vi "CSM to check message.vi"() -> ()   [LabVIEW 2014]
uses:
  user.lib/_NEVSTOP/Communicable State Machine(CSM)/_Support/Priority Queue/Priority Queue.lvclass/Priority Queue.ctl
  user.lib/_NEVSTOP/Communicable State Machine(CSM)/_Support/Process/CSMP-Async Call.vi
  user.lib/_NEVSTOP/Communicable State Machine(CSM)/_Support/GlobalEvent/GEvt-Generate Status Log.vi
  user.lib/_NEVSTOP/Communicable State Machine(CSM)/_Support/Process/CSMP-Broadcast.vi
  user.lib/_NEVSTOP/Communicable State Machine(CSM)/_Support/GlobalEvent/GEvt-Generate Interrupt Log.vi
  user.lib/_NEVSTOP/Communicable State Machine(CSM)/_Support/GlobalEvent/GEvt-Generate Register Log.vi
  user.lib/_NEVSTOP/Communicable State Machine(CSM)/_Support/Process/CSMP-Register Status.vi
  user.lib/_NEVSTOP/Communicable State Machine(CSM)/_Support/GlobalEvent/GEvt-Generate Unregister Log.vi
  user.lib/_NEVSTOP/Communicable State Machine(CSM)/_Support/Process/CSMP-Unregister Status.vi
  user.lib/_NEVSTOP/Communicable State Machine(CSM)/_Support/Process/CSMP-Sync Call.vi
  user.lib/_NEVSTOP/Communicable State Machine(CSM)/_Support/CSMQ/_CSMObj-Unlock.vi
  user.lib/_NEVSTOP/Communicable State Machine(CSM)/_Support/Process/CSMP-PostPostMsg.vi
  user.lib/_NEVSTOP/Communicable State Machine(CSM)/_Support/Process/CSMP-PostSendMsg.vi
  user.lib/_NEVSTOP/Communicable State Machine(CSM)/_Support/CSMQ/_CSMObj-Lock State.vi
  user.lib/_NEVSTOP/Communicable State Machine(CSM)/_Support/Common/Splite Reason String Part.vi
  user.lib/_NEVSTOP/Communicable State Machine(CSM)/_Support/Common/Trim Single line Text.vi
  user.lib/_NEVSTOP/Communicable State Machine(CSM)/_Support/CSMQ/_CSMOFGV Release.vi
  user.lib/_NEVSTOP/Communicable State Machine(CSM)/_Support/Common/Remove Comments from Line.vi
  user.lib/_NEVSTOP/Communicable State Machine(CSM)/_Support/Common/Splite Single-line Message.vi
  user.lib/_NEVSTOP/Communicable State Machine(CSM)/_Support/Common/Parse Next Single-line State.vi
  user.lib/_NEVSTOP/Communicable State Machine(CSM)/_Support/CSMQ/_CSMObj-Log Error if in a Remote Session.vi
  user.lib/_NEVSTOP/Communicable State Machine(CSM)/_Support/CSMQ/_CSMOFGV Obtain.vi
  user.lib/_NEVSTOP/Communicable State Machine(CSM)/_Support/GlobalEvent/GEvt-Generate State Change Log.vi
  user.lib/_NEVSTOP/Communicable State Machine(CSM)/_Support/GlobalEvent/GEvt-Generate Remaining States Log.vi
  user.lib/_NEVSTOP/Communicable State Machine(CSM)/_Support/GlobalEvent/GEvt-Generate Complete Log.vi
  user.lib/_NEVSTOP/Communicable State Machine(CSM)/AdvanceAPI/CSM - Revert Arguments-Safe String.vi
  user.lib/_NEVSTOP/Communicable State Machine(CSM)/_Support/CSMQ/_CSMObj-Message Check.vi
  user.lib/_NEVSTOP/Communicable State Machine(CSM)/_Support/FGV-BroadcastRegistry/Cache-Broadcast Registry Search Result.vi
  user.lib/_NEVSTOP/Communicable State Machine(CSM)/AdvanceAPI/CSM - Register Status Change.vi
  user.lib/_NEVSTOP/Communicable State Machine(CSM)/AdvanceAPI/CSM - Unregister Status Change.vi
  user.lib/_NEVSTOP/Communicable State Machine(CSM)/Utility/uuid.vi
  user.lib/_NEVSTOP/Communicable State Machine(CSM)/_Support/Common/CSM-Name to CSM-Mode.vi
  user.lib/_NEVSTOP/Communicable State Machine(CSM)/_Support/Priority Queue/Not a Refnum.vi
  user.lib/_NEVSTOP/Communicable State Machine(CSM)/AdvanceAPI/CSM - Keywords.vi
  user.lib/_NEVSTOP/Communicable State Machine(CSM)/_Support/GlobalEvent/FGV-GlobalEventRef.vi
  user.lib/_NEVSTOP/Communicable State Machine(CSM)/_Support/CSMQ/_CSMOFGV.vi
  user.lib/_NEVSTOP/Communicable State Machine(CSM)/_Support/CSMQ/_CSMOFGV Dequeue.vi
  user.lib/_NEVSTOP/Communicable State Machine(CSM)/_Support/CSMQ/_CSMObj-Enqueue Cross-Module Message.vi
  user.lib/_NEVSTOP/Communicable State Machine(CSM)/_Support/GlobalEvent/FGV-StatusChangeEventRef.vi
  user.lib/_NEVSTOP/Communicable State Machine(CSM)/_Support/FGV-BroadcastRegistry/global-Broadcast Cache Change Flag.vi
  user.lib/_NEVSTOP/Communicable State Machine(CSM)/_Support/FGV-BroadcastRegistry/FGV-BroadcastRegistry.vi
  user.lib/_NEVSTOP/Communicable State Machine(CSM)/Communicable State Machine.lvlib
panel:
  in  "DoSth: DoB -@ CSM":bool
  in  "DoSth: DoB -> CSM":bool
  in  "DoSth: DoA -@ CSM":bool
  in  "DoSth: DoA -> CSM":bool
  in  "API: API2 -@ CSM":bool
  in  "API: API2 -> CSM":bool
  in  "API: API1 -@ CSM":bool
  in  "API: API1 -> CSM":bool
  out "State History":string
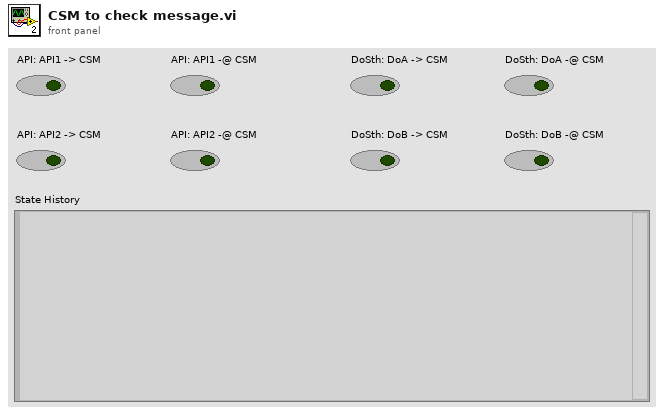
[diagram p1: front panel]
types:
  T1 = enum32{"Invalid", "Standard", "Closed", "Hidden", "Minimized", "Maximized"}
  T2 = enum32{"invalid app kind", "Development System", "Run Time System", "Student Edition", "Embedded LabVIEW", "Evaluation", "Custom"}
  T3 = typedef "Communicable State Machine.lvlib/_CSM_Response Source Message.ctl" = cluster{"‘State":string, "’Arguments":string, "’Error":errorcluster}
  T4 = cluster{"Core":cluster{"Current VI Reference":refnum<vi>, "Close Panel on Exit?":bool}, "Your Boolean data":bool, "Your string data":string}
  T5 = cluster{"Current VI Reference":refnum<vi>, "Close Panel on Exit?":bool}
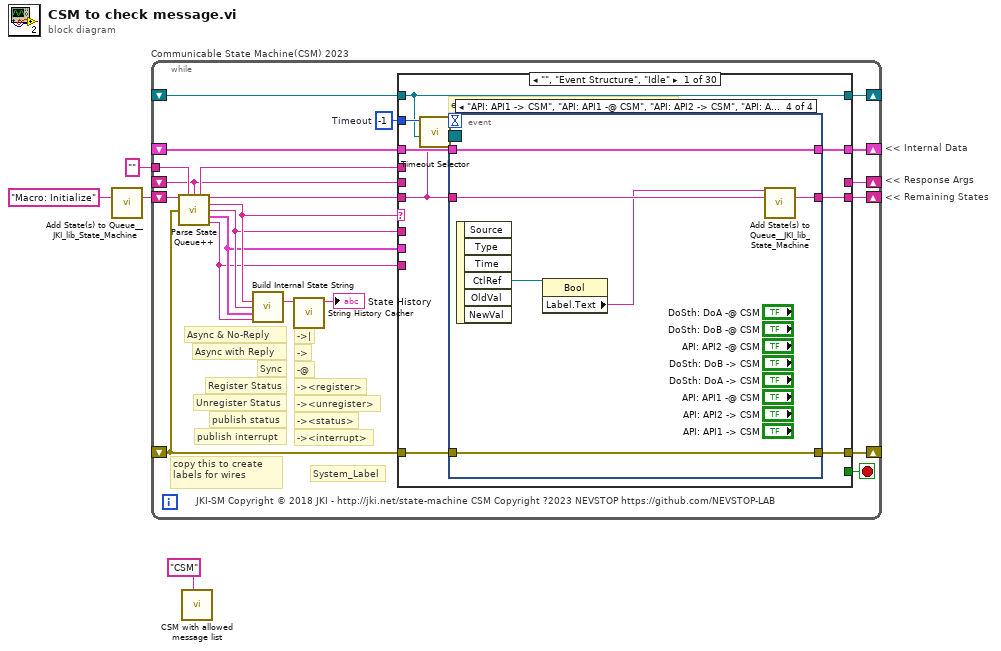
[diagram p0: block diagram]
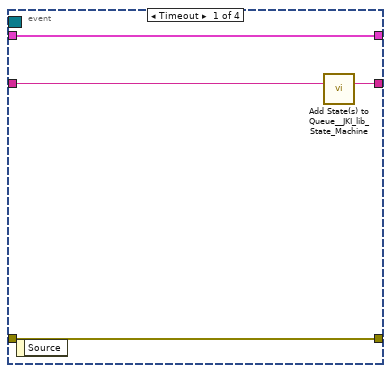
[diagram p2: hidden frame]
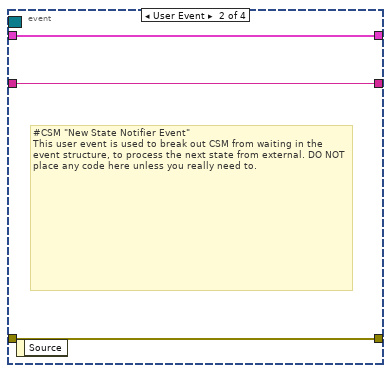
[diagram p3: hidden frame]
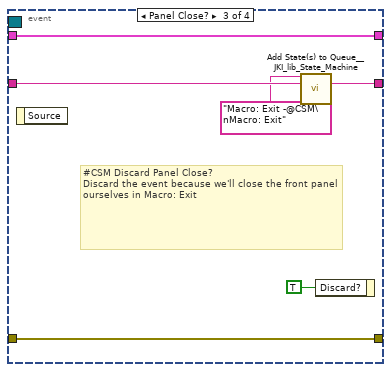
[diagram p4: hidden frame]
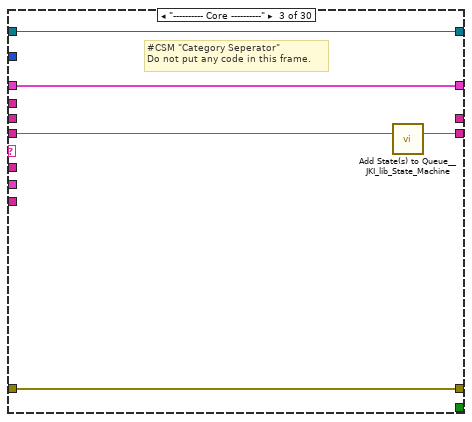
[diagram p6: hidden frame]
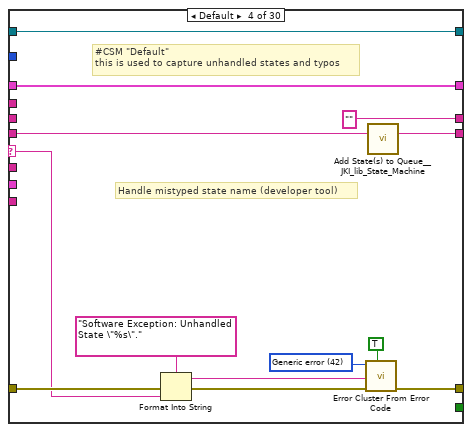
[diagram p7: hidden frame]
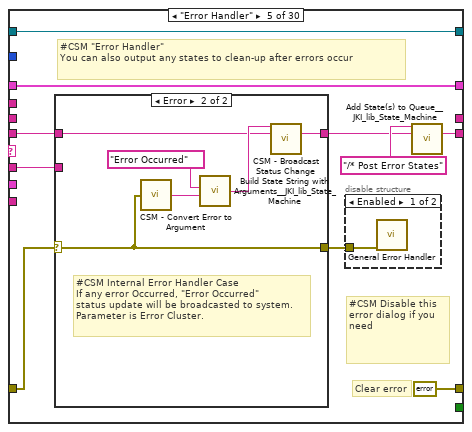
[diagram p8: hidden frame]
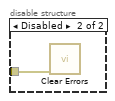
[diagram p9: hidden frame]
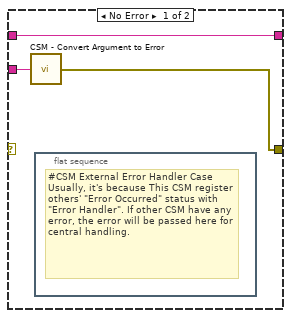
[diagram p10: hidden frame]
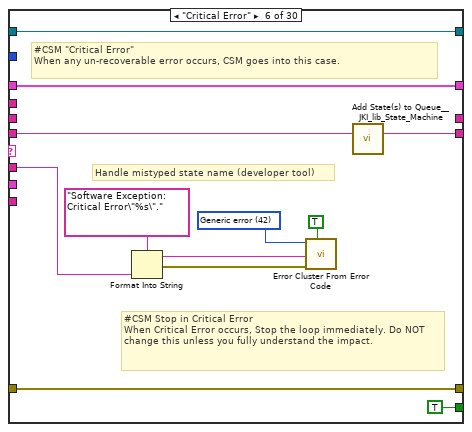
[diagram p11: hidden frame]
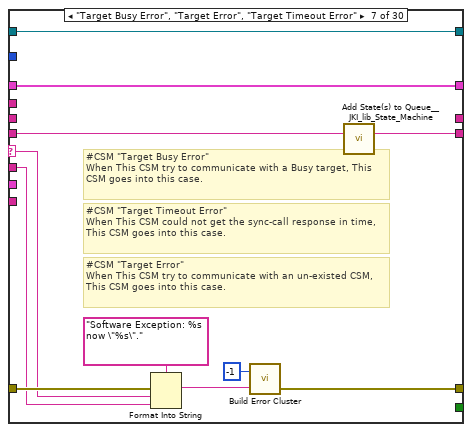
[diagram p12: hidden frame]
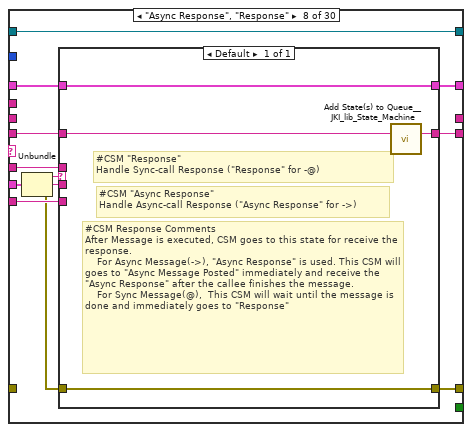
[diagram p13: hidden frame]
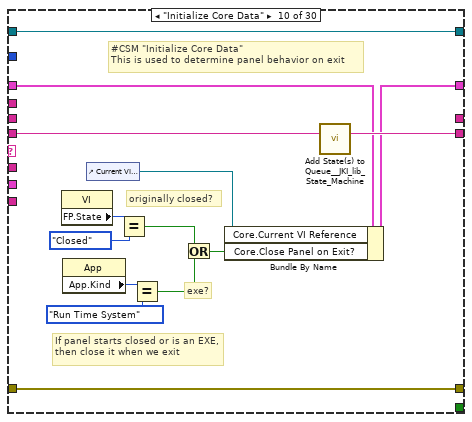
[diagram p15: hidden frame]
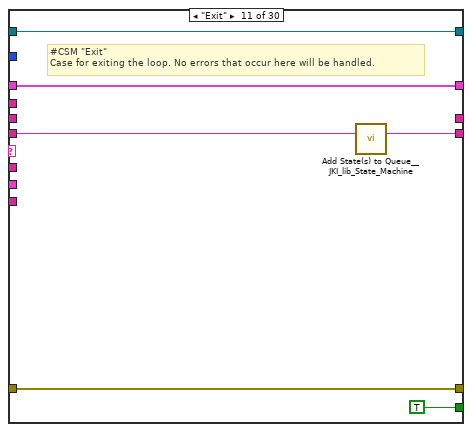
[diagram p16: hidden frame]
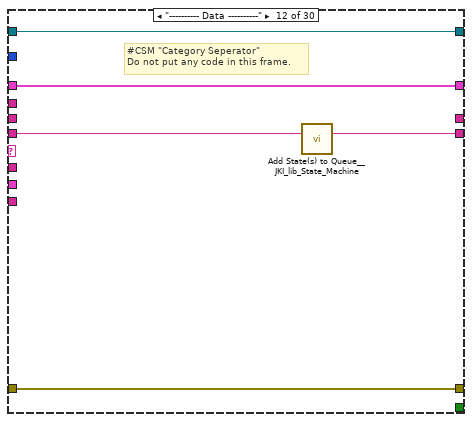
[diagram p17: hidden frame]
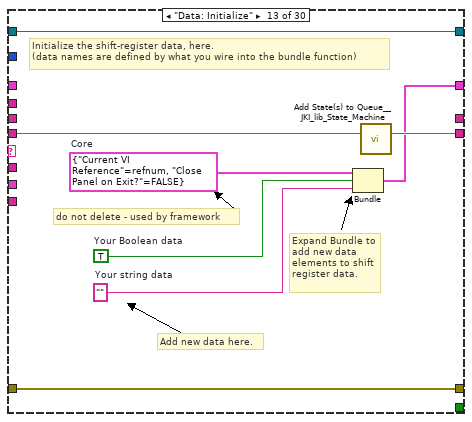
[diagram p18: hidden frame]
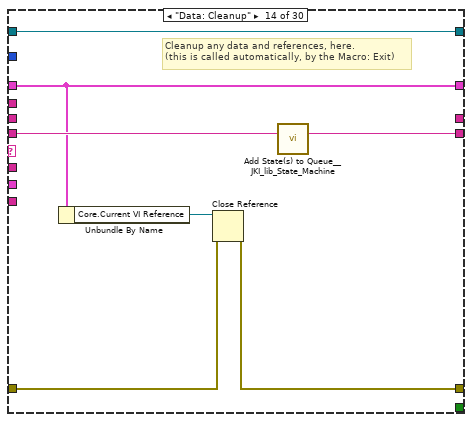
[diagram p19: hidden frame]
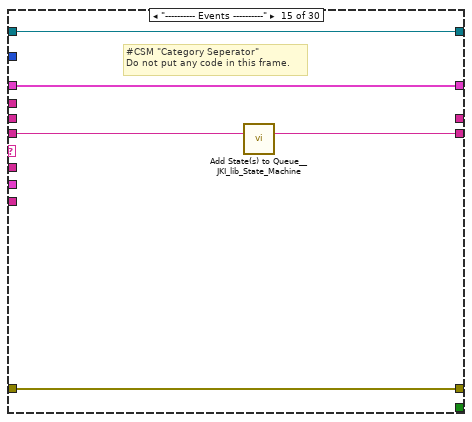
[diagram p20: hidden frame]
diagram:
  # "<< Internal Data"
  # "<< Response Args"
  # "<< Remaining States"
  n1 = call <vilib>:"Add State(s) to Queue__JKI_lib_State_Machine.vi"("State(s) in (\"\")"="Macro: Initialize" ("Init State(\"Macro: Initialize\")")) -> ("States Out"=w4:string)  [unwired: 14 in]
  n2 = while "Communicable State Machine(CSM) 2023" {
    shift-right: [w20] -> _
    shift-left: _ -> [w19]
    shift-right: [w23] -> _
    shift-left: _ -> [w17]
    shift-right: [w22] -> _
    shift-left: w4 -> [w24]
    tunnel: "" ("Name(\"\" to use uuid)") -> [w13]
    shift-right: [w16] -> _
    shift-left: _ -> [w5]
    shift-right: [w15] -> _
    shift-left: _ -> [w14]
    stop <- w21 stop-if-true
    w18 = -1  # Timeout
    # "-><interrupt>"
    # "-><status>"
    # "-><unregister>"
    # "-><register>"
    # "-@"
    # "->"
    # "->|"
    # "publish interrupt"
    # "publish status"
    # "Unregister Status"
    # "Register Status"
    # "Sync"
    # "Async with Reply"
    # "Async & No-Reply"
    # "copy this to create labels for wires"
    # "System_Label"
    # "JKI-SM Copyright © 2018 JKI - http://jki.net/state-machine CSM Copyright ?2023 NEVSTOP https://github.com/NEVSTOP-LAB"
    n3 = call "Parse State Queue++.vi"("State Queue"=w24, "Name(\"\" to use uuid)"=w13, "Response Arguments"=w5, "Error In (no error)"=w17) -> ("Name Used"=w6:string, "Remaining States"=w25:string, "Current State"=w10:string, "Arguments"=w9:string, ">> Response Source Message >>"=w8:T3, ">> Source CSM >>"=w7:string)  [unwired: 6 in]
    n4 = call "Build Internal State String.vi"("State"=w10, "Arguments (\"\")"=w9, ">> Response Source Message >>"=w8, "Source (\"\")"=w7) -> ("State with Arguments"=w11:string)  [unwired: 11 in]
    n5 = call "String History Cacher.vi"("String"=w11) -> ("String Cache"=→"State History":string)  [unwired: 10 in]
    n6 = case shown="\"\", \"Event Structure\", \"Idle\"" w10 {
      selector: w10 -> [_ _ _ w65 _ _ w112 _ _ _ _ _ _ _ _ _ _ _ _ _ _ _ _ _ _ _ _ _ _ _]
      tunnel: w25 -> [w26 w56 w62 w69 w80 w106 w114 w125 w138 w153 w159 w164 w172 w179 w184 w191 w195 w201 w206 w213 w229 w299 w305 w316 w319 w324 w330 w338 w344 w350]
      tunnel: w9 -> [_ _ _ _ w79 w99 w113 w124 _ _ _ _ _ _ _ _ _ _ _ w208 w223 _ _ _ _ _ w327 _ _ _]
      tunnel: w19 -> [w33 w55 w59 w67 w84 w107 w116 w127 w137 w146 w157 w161 _ w174 w181 w190 w194 w198 w204 w211 w225 w296 w302 w313 w318 w323 w329 w335 w341 w347]
      tunnel: [w32 w57 w60 w71 errorcluster {"status"=FALSE, "code"=0, "source"=""} ("error out") w108 w110 w130 w139 w150 w156 w162 w169 w175 w182 w185 w193 w199 w203 w209 w226 w297 w303 w314 w320 w325 w331 w336 w342 w348] -> w23
      tunnel: w17 -> [w31 w57 w60 w70 w81 w108 w118 _ w139 w150 w156 w162 w169 w176 w182 _ w196 w199 w203 w210 w227 w297 w303 w314 w320 w325 w331 w336 w342 w348]
      tunnel: [w34 w56 w61 w68 w76 w105 w117 w126 w138 w152 w158 w163 w171 w178 w183 w191 w195 w200 w205 w212 w228 w298 w304 w315 w319 w324 w330 w337 w343 w349] -> w22
      tunnel: [_ _ _ _ _ TRUE _ _ _ _ TRUE _ _ _ _ _ _ _ _ _ _ _ _ _ _ _ _ _ _ _] -> w21
      tunnel: [w30 w55 w59 w67 w84 w107 w116 w128 w137 w151 w157 w161 w170 w174 w181 w190 w194 w198 w204 w211 w225 w296 w302 w313 w318 w323 w329 w335 w341 w347] -> w20
      tunnel: w18 -> [w29 _ _ _ _ _ _ _ _ _ _ _ _ _ _ _ _ _ _ _ _ _ _ _ _ _ _ _ _ _]
      tunnel: w7 -> [_ _ _ _ _ _ _ w122 _ _ _ _ _ _ _ _ _ _ _ _ _ _ _ _ _ _ _ _ _ _]
      tunnel: w8 -> [_ _ _ _ _ _ _ w129 _ _ _ _ _ _ _ _ _ _ _ _ _ _ _ _ _ _ _ _ _ _]
      tunnel: [_ _ _ "" _ _ _ _ _ _ _ _ _ _ _ _ _ _ _ _ _ _ _ _ _ "API1 Response" w326 _ "DoA Finished" "DoB Finished"] -> w16
      tunnel: [w28 w54 w58 w63 w83 w97 w115 w131 w136 w140 w154 w160 w165 w173 w180 w189 w192 w197 w202 w207 w222 w295 w300 w306 w317 w322 w328 w334 w340 w346] -> w15
      tunnel: w14 -> [w28 w54 w58 w63 w83 w97 w115 w131 w136 w140 w154 w160 w165 w173 w180 _ w192 w197 w202 w207 w222 w295 w300 w306 w317 w322 w328 w334 w340 w346]
      tunnel: w6 -> [_ _ _ _ _ _ _ _ _ _ _ _ _ _ _ w188 _ _ _ _ _ _ _ _ _ _ _ _ _ _]
      tunnel: w5 -> [_ _ _ _ _ _ _ _ _ _ _ _ _ _ _ _ _ _ _ _ _ _ _ _ _ _ _ _ _ _]
      frame "", "Event Structure", "Idle" {
        # "executes when the state queue is empty"
        n7 = call "Timeout Selector.vi"("Remaining States"=w26, "Timeout Expected"=w29) -> ("Timeout"=w27:i32)  [unwired: 5 in]
        n8 = event shown="[3] \"API: API1 -> CSM\", \"API: API1 -@ CSM\", \"API: API2 -> CSM\", \"API: API2 -@ CSM\", \"DoSth: DoA -> CSM\", \"DoSth: DoA -@ CSM\", \"DoSth: DoB -> CSM\", \"DoSth: DoB -@ CSM\": Value Change" {
          selector: w28 -> [_ _ _ _]
          dyn-events: _ -> [_ _ _ _]
          timeout: w27 -> [_ _ _ _]
          tunnel: w26 -> [w38 w40 w47 w51]
          tunnel: [w37 w40 w46 w50] -> w34
          tunnel: w33 -> [w35 w41 w44 w52]
          tunnel: [w36 w39 w45 w53] -> w32
          tunnel: w31 -> [w36 w39 w45 w53]
          tunnel: [w35 w41 w44 w52] -> w30
          event Timeout {
            n9 = event-data() -> ()  [unwired: 1 in, 1 out]
            n10 = call <vilib>:"Add State(s) to Queue__JKI_lib_State_Machine.vi"("State(s) in (\"\")"=w38) -> ("States Out"=w37:string)  [unwired: 14 in]
          }
          event User Event {
            # "#CSM \"New State Notifier Event\"\nThis user event is used to break out CSM from waiting in the event structure, to process the next state from external. DO NOT place any code here unless you really need to."
            n11 = event-data() -> ()  [unwired: 1 in, 1 out]
          }
          event Panel Close? {
            # "#CSM Discard Panel Close?\nDiscard the event because we'll close the front panel ourselves in Macro: Exit"
            n12 = event-data() -> ()  [unwired: 1 in, 1 out]
            n13 = call <vilib>:"Add State(s) to Queue__JKI_lib_State_Machine.vi"("State(s) in Front (\"\")"="Macro: Exit -@CSM\nMacro: Exit", "State(s) in (\"\")"=w47) -> ("States Out"=w46:string)  [unwired: 13 in]
            n14 = event-data("Discard?"=TRUE) -> ()  [unwired: 1 in, 1 out]
          }
          event "API: API1 -> CSM", "API: API1 -@ CSM", "API: API2 -> CSM", "API: API2 -@ CSM", "DoSth: DoA -> CSM", "DoSth: DoA -@ CSM", "DoSth: DoB -> CSM", "DoSth: DoB -@ CSM": Value Change {
            n15 = event-data() -> ("CtlRef"=w49:refnum<vi>)  [unwired: 1 in, 5 out]
            n16 = property class="Bool"(reference=w49) -> ("Label.Text"=w48:string)  [unwired: 1 in, 2 out]
            n17 = call <vilib>:"Add State(s) to Queue__JKI_lib_State_Machine.vi"("State(s) in Front (\"\")"=w48, "State(s) in (\"\")"=w51) -> ("States Out"=w50:string)  [unwired: 13 in]
          }
        }
      }
      frame "CSM Documentation" {
        # "#CSM README FIRST\n\nCSM is a LabVIEW application framework that builds upon JKI State Machine (JKISM). It follows the pattern of JKISM and extends the keywords to describe message communication between CSM modules, including concepts such as Sync-Message, Async-Message, Subscription/Unsubscription of status - essential elements for creating reusable code modules. For more information, please visit the CSM wiki: https://github.com/NEVSTOP-LAB/JKI-State-Machine-Plus-Plus/wiki\n\nFor instructions on JKI State Machine, visit: http://jki.net/state-machine/\nFor information about CSM, visit: https://github.com/NEVSTOP-LAB"
        # "#CSM \"Documentation\"\nCase for holding CSM Documenation"
      }
      frame "---------- Core ----------" {
        # "#CSM \"Category Seperator\"\nDo not put any code in this frame."
        n18 = call <vilib>:"Add State(s) to Queue__JKI_lib_State_Machine.vi"("State(s) in (\"\")"=w62) -> ("States Out"=w61:string)  [unwired: 14 in]
      }
      frame Default {
        w74 = 42 items=["No error", "Argument error", "Memory is full", "Out of zone", "End of file", "File already open", "Generic file I/O error", "File not found", "File permission error", "Disk is full", "Duplicate path", "Too many files open", "System feature not enabled", "Resource file not found", "Cannot add resource", "Resource not found", "Image not found", "Image memory error", "Pen does not exist", "Config type invalid", "Config token not found", "Config parse error", "Config memory error", "Bad external code format", "Bad external code offset", "External code not present", "Null window", "Destroy window error", "Null menu", "Print aborted", "Bad print record", "Print driver error", "Windows error during printing", "Memory error during printing", "Print dialog error", "Generic print error", "Invalid device refnum", "Device not found", "Device parameter error", "Device unit error", "Cannot open device", "Device call aborted", "Generic error", "Cancelled by user", "Object ID too low", "Object ID too high", "Object not in heap", "Unknown heap", "Unknown object (invalid DefProc)", "Unknown object (DefProc not in table)", "Message out of range", "Invalid (null) method", "Unknown message", "Manager call not supported", "Bad address", "Network operation in progress", "Network operation timed out", "Connection is busy", "Network attribute not supported", "Network error", "Address in use", "System out of memory", "Connection aborted", "Connection refused", "Not connected", "Already connected", "Connection closed", "Initialization error (interapplication manager)", "Bad occurrence", "Wait on unbound occurrence handler", "Occurrence queue overflow", "Datalog type conflict", "Unused", "Unrecognized type (interapplication manager)", "Memory corrupt", "Failed to make temporary DLL", "Old CIN version", "Drag socket not found", "Failed to load drop-object", "Failed to register OLE object", "Failed to release OLE object", "Format specifier type mismatch", "Unknown format specifier", "Too few format specifiers", "Too many format specifiers", "Scan failed", "Newer CIN version", "Error converting to variant", "Runtime menu error", "Password tampered", "Variant attribute not found", "Incompatible variant data type", "Event data is not available", "Event Store is not present", "Occurrence is not found", "Event Queue is not created", "Event info is not available", "Refnum passed is NULL", "Error retrieving Class GUID", "Error retrieving CoClass GUID", "Error retrieving TypeLib GUID.", "Bad built application magic bytes.", "Specific driver is different from the specific driver associated with the Logical Name.", "There is no session opened to the class driver.", "Max Error", "MAX - Error with config objects", "MAX - Error loading configuration", "MAX - Group not supported"]
        # "#CSM \"Default\"\nthis is used to capture unhandled states and typos"
        # "Handle mistyped state name (developer tool)"
        n19 = Format Into String(format string="Software Exception: Unhandled State \"%s\"." ("message"), error in=w70, w65) -> (resulting string=w73:string, error out=w72:errorcluster)  [unwired: 1 in]
        n20 = call <vilib>:"Error Cluster From Error Code.vi"("show call chain? (False)"=TRUE, "error in (no error)"=w72, "error message (\"\")"=w73, "error code (0)"=w74) -> ("error out"=w71:errorcluster)  [unwired: 5 in]
        n21 = call <vilib>:"Add State(s) to Queue__JKI_lib_State_Machine.vi"("State(s) in (\"\")"=w69) -> ("States Out"=w68:string)  [unwired: 14 in]
      }
      frame "Error Handler" {
        # "#CSM Disable this error dialog if you need"
        # "#CSM \"Error Handler\"\nYou can also output any states to clean-up after errors occur"
        # "Clear error"
        n22 = case shown="Error" w81 {
          selector: w81 -> [_ w91]
          tunnel: [w90 w93] -> w77
          tunnel: w80 -> [w90 w92]
          tunnel: w79 -> [w89 _]
          tunnel: [w88 w91] -> w82
          frame No Error {
            n23 = call "CSM - Convert Argument to Error.vi"("Argument"=w89) -> ("error"=w88:errorcluster)  [unwired: 4 in]
            n24 = flat-sequence {
              frame #0 {
                # "#CSM External Error Handler Case\nUsually, it's because This CSM register others' \"Error Occurred\" status with \"Error Handler\". If other CSM have any error, the error will be passed here for central handling."
              }
            }
          }
          frame Error {
            # "#CSM Internal Error Handler Case \nIf any error Occurred, \"Error Occurred\" \nstatus update will be broadcasted to system.\nParameter is Error Cluster."
            n25 = call "CSM - Convert Error to Argument.vi"("error in (no error)"=w91) -> ("Arguments"=w95:string)  [unwired: 4 in]
            n26 = call <vilib>:"Build State String with Arguments__JKI_lib_State_Machine.vi"("Arguments (\"\")"=w95, "State"="Error Occurred" ("Status with Arguments")) -> ("State with Arguments"=w94:string)  [unwired: 4 in]
            n27 = call "CSM - Broadcast Status Change.vi"("Status with Arguments"=w94, "State Queue"=w92) -> ("Remaining States"=w93:string)  [unwired: 13 in]
          }
        }
        n28 = disable-structure shown="Enabled" {
          disable-tunnel: w82 -> [w86 w87]
          frame Enabled {
            n29 = call <vilib>:"General Error Handler.vi"("error in (no error)"=w86) -> ()  [unwired: 10 in, 5 out]
          }
          frame Disabled {
            n30 = call <vilib>:"Clear Errors.vi"("error in (no error)"=w87) -> ()  [unwired: 6 in, 1 out]
          }
        }
        n31 = call <vilib>:"Add State(s) to Queue__JKI_lib_State_Machine.vi"("State(s) in Front (\"\")"="/* Post Error States", "State(s) in (\"\")"=w77) -> ("States Out"=w76:string)  [unwired: 13 in]
      }
      frame "Critical Error" {
        w103 = 42 items=["No error", "Argument error", "Memory is full", "Out of zone", "End of file", "File already open", "Generic file I/O error", "File not found", "File permission error", "Disk is full", "Duplicate path", "Too many files open", "System feature not enabled", "Resource file not found", "Cannot add resource", "Resource not found", "Image not found", "Image memory error", "Pen does not exist", "Config type invalid", "Config token not found", "Config parse error", "Config memory error", "Bad external code format", "Bad external code offset", "External code not present", "Null window", "Destroy window error", "Null menu", "Print aborted", "Bad print record", "Print driver error", "Windows error during printing", "Memory error during printing", "Print dialog error", "Generic print error", "Invalid device refnum", "Device not found", "Device parameter error", "Device unit error", "Cannot open device", "Device call aborted", "Generic error", "Cancelled by user", "Object ID too low", "Object ID too high", "Object not in heap", "Unknown heap", "Unknown object (invalid DefProc)", "Unknown object (DefProc not in table)", "Message out of range", "Invalid (null) method", "Unknown message", "Manager call not supported", "Bad address", "Network operation in progress", "Network operation timed out", "Connection is busy", "Network attribute not supported", "Network error", "Address in use", "System out of memory", "Connection aborted", "Connection refused", "Not connected", "Already connected", "Connection closed", "Initialization error (interapplication manager)", "Bad occurrence", "Wait on unbound occurrence handler", "Occurrence queue overflow", "Datalog type conflict", "Unused", "Unrecognized type (interapplication manager)", "Memory corrupt", "Failed to make temporary DLL", "Old CIN version", "Drag socket not found", "Failed to load drop-object", "Failed to register OLE object", "Failed to release OLE object", "Format specifier type mismatch", "Unknown format specifier", "Too few format specifiers", "Too many format specifiers", "Scan failed", "Newer CIN version", "Error converting to variant", "Runtime menu error", "Password tampered", "Variant attribute not found", "Incompatible variant data type", "Event data is not available", "Event Store is not present", "Occurrence is not found", "Event Queue is not created", "Event info is not available", "Refnum passed is NULL", "Error retrieving Class GUID", "Error retrieving CoClass GUID", "Error retrieving TypeLib GUID.", "Bad built application magic bytes.", "Specific driver is different from the specific driver associated with the Logical Name.", "There is no session opened to the class driver.", "Max Error", "MAX - Error with config objects", "MAX - Error loading configuration", "MAX - Group not supported"]
        # "#CSM Stop in Critical Error\nWhen Critical Error occurs, Stop the loop immediately. Do NOT change this unless you fully understand the impact."
        # "#CSM \"Critical Error\"\nWhen any un-recoverable error occurs, CSM goes into this case."
        # "Handle mistyped state name (developer tool)"
        n32 = Format Into String(format string="Software Exception: Critical Error\"%s\"." ("message"), w99) -> (resulting string=w102:string, error out=w101:errorcluster)  [unwired: 2 in]
        n33 = call <vilib>:"Error Cluster From Error Code.vi"("show call chain? (False)"=TRUE, "error in (no error)"=w101, "error message (\"\")"=w102, "error code (0)"=w103) -> ()  [unwired: 5 in, 1 out]
        n34 = call <vilib>:"Add State(s) to Queue__JKI_lib_State_Machine.vi"("State(s) in (\"\")"=w106) -> ("States Out"=w105:string)  [unwired: 14 in]
      }
      frame "Target Busy Error", "Target Error", "Target Timeout Error" {
        # "#CSM \"Target Error\"\nWhen This CSM try to communicate with an un-existed CSM, This CSM goes into this case."
        # "#CSM \"Target Timeout Error\"\nWhen This CSM could not get the sync-call response in time, This CSM goes into this case."
        # "#CSM \"Target Busy Error\"\nWhen This CSM try to communicate with a Busy target, This CSM goes into this case."
        n35 = Format Into String(format string="Software Exception: %s now \"%s\"." ("message"), error in=w118, w112, w113) -> (resulting string=w111:string)  [unwired: 1 in, 1 out]
        n36 = call "Build Error Cluster.vi"("String to Prepend to source (\"\")"=w111, "code"=-1) -> ("error out"=w110:errorcluster)
        n37 = call <vilib>:"Add State(s) to Queue__JKI_lib_State_Machine.vi"("State(s) in (\"\")"=w114) -> ("States Out"=w117:string)  [unwired: 14 in]
      }
      frame "Async Response", "Response" {
        n38 = Unbundle(w129) -> ("‘State"=w123:string, "’Arguments"=w121:string, "’Error"=w120:errorcluster)
        n39 = case shown="Default" w123 {
          tunnel: [w135] -> w130
          tunnel: w120 -> [w135]
          tunnel: [w134] -> w128
          tunnel: w127 -> [w134]
          tunnel: [w132] -> w126
          tunnel: w125 -> [w133]
          tunnel: w124 -> [_]
          tunnel: w122 -> [_]
          tunnel: w121 -> [_]
          frame Default {
            # "#CSM Response Comments\nAfter Message is executed, CSM goes to this state for receive the response.\n    For Async Message(->), \"Async Response\" is used. This CSM will goes to \"Async Message Posted\" immediately and receive the \"Async Response\" after the callee finishes the message.\n    For Sync Message(@),  This CSM will wait until the message is done and immediately goes to \"Response\""
            # "#CSM \"Async Response\"\nHandle Async-call Response (\"Async Response\" for ->)"
            # "#CSM \"Response\"\nHandle Sync-call Response (\"Response\" for -@)"
            n40 = call <vilib>:"Add State(s) to Queue__JKI_lib_State_Machine.vi"("State(s) in (\"\")"=w133) -> ("States Out"=w132:string)  [unwired: 14 in]
          }
        }
      }
      frame "Async Message Posted" {
        # "#CSM \"Async Message Posted\"\nAfter Async Message is posted (-> or ->| ), CSM goes to this state for post-action.\nYou can use Argument - State to tell which Async Message is called."
      }
      frame "Initialize Core Data" {
        # "#CSM \"Initialize Core Data\"\nThis is used to determine panel behavior on exit"
        # "originally closed?"
        # "exe?"
        # "If panel starts closed or is an EXE, then close it when we exit"
        n41 = property class="VI"() -> ("FP.State"=w143:T1)  [unwired: 2 in, 2 out]
        n42 = property class="App"() -> ("App.Kind"=w149:T2)  [unwired: 2 in, 2 out]
        n43 = control-ref of="Current VI Reference"() -> (w144:refnum<vi>)
        n44 = Equal?(x=w143, y=T1."Closed" ("Front Panel Window:State")) -> (x = y?=w141:bool)
        n45 = Equal?(x=w149, y=T2."Run Time System" ("Application:Kind")) -> (x = y?=w147:bool)
        n46 = Or(x=w141, y=w147) -> (x .or. y?=w145:bool)
        n47 = Bundle By Name(cluster=w146, "Core.Current VI Reference"=w144, "Core.Close Panel on Exit?"=w145) -> (w151:T4)
        n48 = call <vilib>:"Add State(s) to Queue__JKI_lib_State_Machine.vi"("State(s) in (\"\")"=w153) -> ("States Out"=w152:string)  [unwired: 14 in]
      }
      frame "Exit" {
        # "#CSM \"Exit\"\nCase for exiting the loop. No errors that occur here will be handled."
        n49 = call <vilib>:"Add State(s) to Queue__JKI_lib_State_Machine.vi"("State(s) in (\"\")"=w159) -> ("States Out"=w158:string)  [unwired: 14 in]
      }
      frame "---------- Data ----------" {
        # "#CSM \"Category Seperator\"\nDo not put any code in this frame."
        n50 = call <vilib>:"Add State(s) to Queue__JKI_lib_State_Machine.vi"("State(s) in (\"\")"=w164) -> ("States Out"=w163:string)  [unwired: 14 in]
      }
      frame "Data: Initialize" {
        w166 = T5 {"Current VI Reference"=refnum, "Close Panel on Exit?"=FALSE}  # Core
        w168 = TRUE  # Your Boolean data
        w167 = ""  # Your string data
        # "do not delete - used by framework"
        # "Expand Bundle to add new data elements to shift register data."
        # "Add new data here."
        # "Initialize the shift-register data, here.\n(data names are defined by what you wire into the bundle function)"
        n51 = Bundle("Core"=w166, "Your Boolean data"=w168, "Your string data"=w167) -> (w170:T4)  [unwired: 1 in]
        n52 = call <vilib>:"Add State(s) to Queue__JKI_lib_State_Machine.vi"("State(s) in (\"\")"=w172) -> ("States Out"=w171:string)  [unwired: 14 in]
      }
      frame "Data: Cleanup" {
        # "Cleanup any data and references, here.\n(this is called automatically, by the Macro: Exit)"
        n53 = Unbundle By Name(w174) -> ("Core.Current VI Reference"=w177:refnum<vi>)
        n54 = Close Reference(reference=w177, error in (no error)=w176) -> (error out=w175:errorcluster)
        n55 = call <vilib>:"Add State(s) to Queue__JKI_lib_State_Machine.vi"("State(s) in (\"\")"=w179) -> ("States Out"=w178:string)  [unwired: 14 in]
      }
      frame "---------- Events ----------" {
        # "#CSM \"Category Seperator\"\nDo not put any code in this frame."
        n56 = call <vilib>:"Add State(s) to Queue__JKI_lib_State_Machine.vi"("State(s) in (\"\")"=w184) -> ("States Out"=w183:string)  [unwired: 14 in]
      }
      frame "Events: Register" {
        # "#CSM \"Events: Register\"\nRegister user event. New Message Event is registered to break CSM waiting in event structure by default."
        # "#CSM Register New Message Event\nRegister message event to break Waiting in Event structure."
        n57 = call "CSM - Get New State Notifier Event.vi"("Name(\"\" to use uuid) in"=w188) -> ("Error out"=w186:errorcluster, "New State Notifier Event"=w187:refnum<user-event>)  [unwired: 9 in]
        n58 = register-events(error in=w186, w187) -> (reference out=w189:refnum<event-registration>, error out=w185:errorcluster)  [unwired: 1 in]
      }
      frame "Events: Unregister" {
        # "#CSM \"Events: Unregister\"\nUnregister user event."
        n59 = Unregister For Events(event registration refnum=w192, error in=w196) -> (error out=w193:errorcluster)
      }
      frame "---------- UI ----------" {
        # "#CSM \"Category Seperator\"\nDo not put any code in this frame."
        n60 = call <vilib>:"Add State(s) to Queue__JKI_lib_State_Machine.vi"("State(s) in (\"\")"=w201) -> ("States Out"=w200:string)  [unwired: 14 in]
      }
      frame "UI: Initialize" {
        # "#CSM \"UI: Initialize\"\nInitialize the User Interface, here.\n(this is called automatically, by the Macro: Init)"
        n61 = call <vilib>:"Add State(s) to Queue__JKI_lib_State_Machine.vi"("State(s) in (\"\")"=w206) -> ("States Out"=w205:string)  [unwired: 14 in]
      }
      frame "UI: Cursor Set" {
        # "#CSM \"UI: Cursor Set\"\nSet and Unset Cursor Busy.\n(Usage: \"UI: Cursor Set >> Busy|Idle\")"
        # "Argument"
        n62 = disable-structure shown="TARGET_TYPE!=Windows" {
          disable-tunnel: w210 -> [w216 w221]
          disable-tunnel: [w215 w221] -> w209
          disable-tunnel: w208 -> [w214 _]
          frame condition #0 (active) {
            n63 = case shown="\"Idle\", Default" w214 {
              tunnel: w216 -> [w218 w220]
              tunnel: [w217 w219] -> w215
              frame "Idle", Default {
                n64 = call <vilib>:"Unset Busy.vi"("error in (no error)"=w218) -> ("error out"=w217:errorcluster)  [unwired: 10 in]
              }
              frame "Busy" {
                n65 = call <vilib>:"Set Busy.vi"("error in (no error)"=w220) -> ("error out"=w219:errorcluster)  [unwired: 9 in, 1 out]
              }
            }
          }
          frame condition #1 {
          }
        }
        n66 = call <vilib>:"Add State(s) to Queue__JKI_lib_State_Machine.vi"("State(s) in (\"\")"=w213) -> ("States Out"=w212:string)  [unwired: 14 in]
      }
      frame "UI: Front Panel State" {
        # "#CSM \"UI: Front Panel State\"\nSet Front Panel Open or Closed\n(Usage: \"UI: Front Panel State >> Open|Close\")"
        # "Argument"
        n67 = Unbundle By Name(w225) -> ("Core.Current VI Reference"=w224:refnum<vi>)
        n68 = call <vilib>:"Add State(s) to Queue__JKI_lib_State_Machine.vi"("State(s) in (\"\")"=w229) -> ("States Out"=w228:string)  [unwired: 14 in]
        n69 = case shown="\"Close\", \"Closed\"" w223 {
          tunnel: w227 -> [w235 w250 w261 w274 w287]
          tunnel: [w237 w251 w263 w276 w289] -> w226
          tunnel: w224 -> [w236 w248 w262 w275 w288]
          frame "Open", "Standard", Default {
            w230 = T1."Standard" ("State")
            n70 = property class="VI"(reference=w236, error in=w235) -> (reference out=w233:refnum<vi>, error out=w234:errorcluster, "FP.State"=w232:T1)
            n71 = Not Equal?(x=w232, y=w230) -> (x != y?=w231:bool)
            n72 = case shown="True" w231 {
              tunnel: [w241 w243] -> w237
              tunnel: w234 -> [w240 w243]
              tunnel: w233 -> [w239 _]
              tunnel: w230 -> [w238 _]
              frame True {
                n73 = invoke class="VI" method="FP.Open"(reference=w239, error in=w240, "Activate"=TRUE, "State"=w238) -> (error out=w241:errorcluster)  [unwired: 1 in, 4 out]
              }
              frame False {
              }
            }
          }
          frame "Close", "Closed" {
            n74 = property class="VI"(reference=w248, error in=w250) -> (reference out=w247:refnum<vi>, error out=w249:errorcluster, "FP.State"=w245:T1)
            n75 = Not Equal?(x=w245, y=T1."Closed" ("Front Panel Window:State")) -> (x != y?=w244:bool)
            n76 = case shown="False" w244 {
              tunnel: [w252 w255] -> w251
              tunnel: w249 -> [w252 w254]
              tunnel: w247 -> [_ w253]
              frame False {
              }
              frame True {
                n77 = invoke class="VI" method="FP.Close"(reference=w253, error in=w254) -> (error out=w255:errorcluster)  [unwired: 1 in, 2 out]
              }
            }
          }
          frame "Hidden", "Hide" {
            w256 = T1."Hidden" ("State")
            n78 = property class="VI"(reference=w262, error in=w261) -> (reference out=w259:refnum<vi>, error out=w260:errorcluster, "FP.State"=w258:T1)
            n79 = Not Equal?(x=w258, y=w256) -> (x != y?=w257:bool)
            n80 = case shown="True" w257 {
              tunnel: [w267 w268] -> w263
              tunnel: w260 -> [w266 w268]
              tunnel: w259 -> [w265 _]
              tunnel: w256 -> [w264 _]
              frame True {
                n81 = invoke class="VI" method="FP.Open"(reference=w265, error in=w266, "State"=w264) -> (error out=w267:errorcluster)  [unwired: 2 in, 4 out]
              }
              frame False {
              }
            }
          }
          frame "Minimize", "Minimized" {
            w269 = T1."Minimized" ("State")
            n82 = property class="VI"(reference=w275, error in=w274) -> (reference out=w272:refnum<vi>, error out=w273:errorcluster, "FP.State"=w271:T1)
            n83 = Not Equal?(x=w271, y=w269) -> (x != y?=w270:bool)
            n84 = case shown="True" w270 {
              tunnel: [w280 w281] -> w276
              tunnel: w273 -> [w279 w281]
              tunnel: w272 -> [w278 _]
              tunnel: w269 -> [w277 _]
              frame True {
                n85 = invoke class="VI" method="FP.Open"(reference=w278, error in=w279, "State"=w277) -> (error out=w280:errorcluster)  [unwired: 2 in, 4 out]
              }
              frame False {
              }
            }
          }
          frame "Maximize", "Maximized" {
            w282 = T1."Maximized" ("State")
            n86 = property class="VI"(reference=w288, error in=w287) -> (reference out=w285:refnum<vi>, error out=w286:errorcluster, "FP.State"=w284:T1)
            n87 = Not Equal?(x=w284, y=w282) -> (x != y?=w283:bool)
            n88 = case shown="True" w283 {
              tunnel: [w293 w294] -> w289
              tunnel: w286 -> [w292 w294]
              tunnel: w285 -> [w291 _]
              tunnel: w282 -> [w290 _]
              frame True {
                n89 = invoke class="VI" method="FP.Open"(reference=w291, error in=w292, "State"=w290) -> (error out=w293:errorcluster)  [unwired: 2 in, 4 out]
              }
              frame False {
              }
            }
          }
        }
      }
      frame "---------- Macro ----------" {
        # "#CSM \"Category Seperator\"\nDo not put any code in this frame."
        n90 = call <vilib>:"Add State(s) to Queue__JKI_lib_State_Machine.vi"("State(s) in (\"\")"=w299) -> ("States Out"=w298:string)  [unwired: 14 in]
      }
      frame "Macro: Initialize" {
        w301 = "Data: Initialize\nInitialize Core Data\nEvents: Register\nUI: Initialize\nUI: Front Panel State >> Open"  # Data: Initialize Initialize Core Data Events: Register UI: Initialize UI: Front Panel State >> Open
        # "#CSM \"Macro: Initialize\"\nInitialization Macro (This is called once, when the VI starts)"
        n91 = call <vilib>:"Add State(s) to Queue__JKI_lib_State_Machine.vi"("State(s) in Front (\"\")"=w301, "State(s) in (\"\")"=w305) -> ("States Out"=w304:string)  [unwired: 13 in]
      }
      frame "Macro: Exit" {
        # "#CSM \"Macro: Exit\"\nExit Macro (This is called once, when the VI exits)"
        n92 = Unbundle By Name(w313) -> ("Core.Close Panel on Exit?"=w312:bool)
        n93 = Select(t="UI: Front Panel State >> Close", s=w312, f="") -> (s? t:f=w309:string)
        n94 = call <vilib>:"Add State(s) to Queue__JKI_lib_State_Machine.vi"("State(s) in (\"\")"=w309, "State(s) at Back (\"\")"="Data: Cleanup\nEvents: Unregister\nExit") -> ("States Out"=w307:string)  [unwired: 13 in]
        n95 = call <vilib>:"Add State(s) to Queue__JKI_lib_State_Machine.vi"("State(s) in Front (\"\")"=w307, "State(s) in (\"\")"=w316) -> ("States Out"=w315:string)  [unwired: 13 in]
      }
      frame "---------- API ----------" {
        # "#CSM \"Category Seperator\"\nDo not put any code in this frame."
      }
      frame "API: API1" {
        # "#CSM API Example\nCopy/Rename this case for your own API"
        # "#CSM Response\nConnect this to return the response of your API"
        # "#CSM >> Source CSM >>\nIf you need to tell who triggered this state , use this string. If it's this case itself, this string is \"\"."
        # "#CSM >> Arguments >>\nDeal with the parameter if any"
      }
      frame "API: API2" {
        # "#CSM API Example\nCopy/Rename this case for your own API"
        # "unpack Hex String  to Variant\nif complex parameter is needed."
        n96 = call "CSM - Convert HexStr to Data.vi"("HEX String"=w327) -> ()  [unwired: 7 in, 2 out]
        n97 = disable-structure shown="Disabled" {
          disable-tunnel: [w332 "API2 Response"] -> w326
          frame Disabled {
            # "pack variant to hexstr \nif complex response is needed."
            # "complex Response"
            n98 = call "CSM - Convert Data to HexStr.vi"() -> ("HEX String (0-9,A-F)"=w332:string)  [unwired: 9 in]
          }
          frame Enabled {
          }
        }
      }
      frame "---------- DoSth ----------" {
        # "#CSM \"Category Seperator\"\nDo not put any code in this frame."
        n99 = call <vilib>:"Add State(s) to Queue__JKI_lib_State_Machine.vi"("State(s) in (\"\")"=w338) -> ("States Out"=w337:string)  [unwired: 14 in]
      }
      frame "DoSth: DoA" {
        # "#CSM \"Internal State\"\nThis category is used for holding internal states"
        n100 = call <vilib>:"Add State(s) to Queue__JKI_lib_State_Machine.vi"("State(s) in (\"\")"=w344) -> ("States Out"=w343:string)  [unwired: 14 in]
      }
      frame "DoSth: DoB" {
        # "#CSM \"Internal State\"\nThis category is used for holding internal states"
        n101 = call <vilib>:"Add State(s) to Queue__JKI_lib_State_Machine.vi"("State(s) in (\"\")"=w350) -> ("States Out"=w349:string)  [unwired: 14 in]
      }
    }
  }
  n102 = call "CSM with allowed message list.vi"("Name(\"\" to use uuid)"="CSM" ("Name(\"\" to use uuid)")) -> ()  [unwired: 11 in]
